vi "sawtooth.vi"(4 "ktrap":sgl, 8 "mobX(px/V)":sgl, 9 "SP_X":sgl, 10 "Xpx":sgl, 11 "Force_ST":sgl) -> (3 "counter Force":sgl)   [LabVIEW 2019]
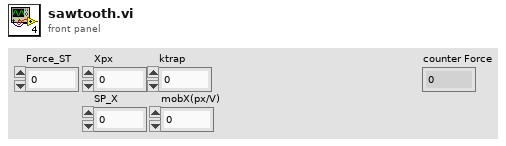
[diagram p1: front panel]
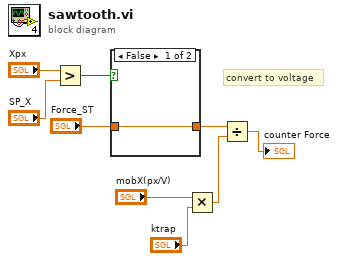
[diagram p0: block diagram]
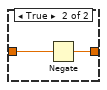
[diagram p2: hidden frame]
diagram:
  # "convert to voltage"
  n1 = Greater?(x="Xpx", y="SP_X") -> (0:w5:bool)
  n2 = case shown="False" w5 {
    tunnel: [w10 w11] -> w1
    tunnel: "Force_ST" -> [w10 w12]
    frame False {
    }
    frame True {
      n3 = Negate(x=w12) -> (-x=w11:sgl)
    }
  }
  n4 = Multiply(x="mobX(px/V)", y="ktrap") -> (x*y=w7:sgl)
  n5 = Divide(x=w1, y=w7) -> (x/y=→"counter Force":sgl)
